vi "纳清蓝绿藻电极校准.vi"() -> ()   [LabVIEW 2016, in "斯坦道多参数.lvlib"]
uses:
  <vilib>/Utility/miscctls.llb/LVPointTypeDef.ctl
  <vilib>/Utility/miscctls.llb/LVPositionTypeDef.ctl
  <vilib>/Analysis/NI_AALBase.lvlib
panel:
  out "第三点信号值":dbl
  out "第二点信号值":dbl
  out "第一点信号值":dbl
  out "报警信息":string
  out "通讯状态":string
  out "第三点校准值":dbl
  out "标液3":sgl
  out "第二点校准值":dbl
  out "第一点校准值":dbl
  in  "校准停止":bool
  in  "校准启动":bool
  in  "校准模式":enum16{"两点校准", "单点校准", "三点校准"}(ring)=enum."单点校准"
  out "最小值":sgl format="%#.2f"
  out "最大值":sgl format="%#.2f"
  out "波形图表":u16(graph) caption="历史曲线"
  out "mean":dbl caption="均值" format="%#.2f"
  out "standard deviation":dbl caption="标准差" format="%#.2f"
  out "变异系数":dbl format="%#.6f"
  out "测量值":sgl format="%#.2f"
  out "提示":string
  out "标液2":sgl
  out "标液1":sgl
  out "原始光强数值":u16 caption="信号值"
  out "温度":dbl format="%#.2f"
  # "藻密度电极设定"
  # "℃"
  # "cells/mL"
  # "请选择校准模式:"
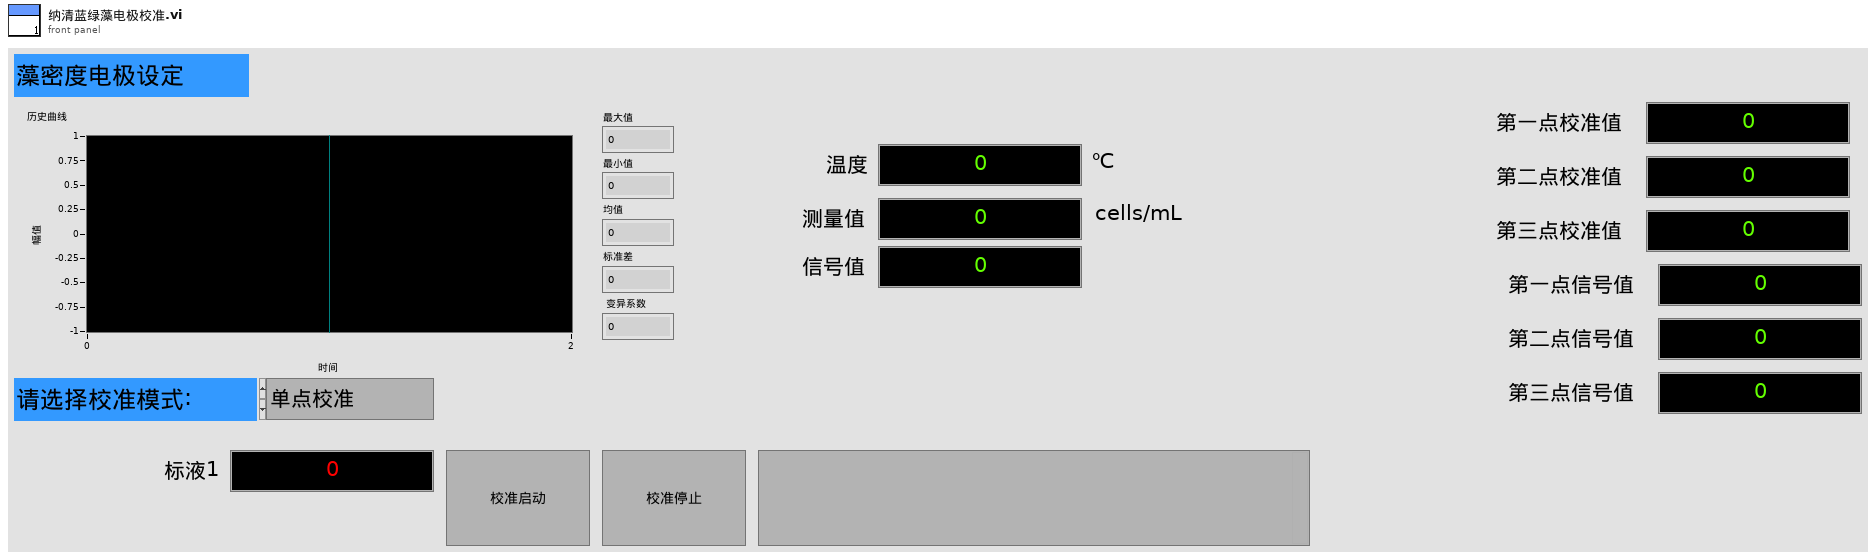
[diagram p1: front panel]
types:
  T1 = typedef "LVPointTypeDef.ctl" = cluster{"Horizontal":i16, "Vertical":i16}
  T2 = cluster{"报警码":u16, "蓝绿藻":sgl, "温度数据":sgl, "原始光强数值":u16, "0X0006_NC":u16, "平均次数":u16, "清扫模式":u16, "清扫次数":u16, "清扫间隔分钟":u16, "0X000B_NC":string, "产品名称":string, "序列号":string, "硬件版本":string, "软件版本":string, "通讯地址":u16, "波特率":u16, "设备类型":u16, "0X0026_NC":string, "0X0030_NC":u16, "第一点原始光强":u16, "第一点校准数据":sgl, "第二点原始光强":u16, "第二点校准数据":sgl, "第三点原始光强":u16, "第三点校准数据":sgl, "探头校准命令":u16, "温度校准参数":sgl, "温度校准命令":u16}
  T3 = typedef "LVPositionTypeDef.ctl" = cluster{"Left":i32, "Top":i32}
  T4 = enum8{"Enabled", "Disabled", "Disabled and Grayed Out"}
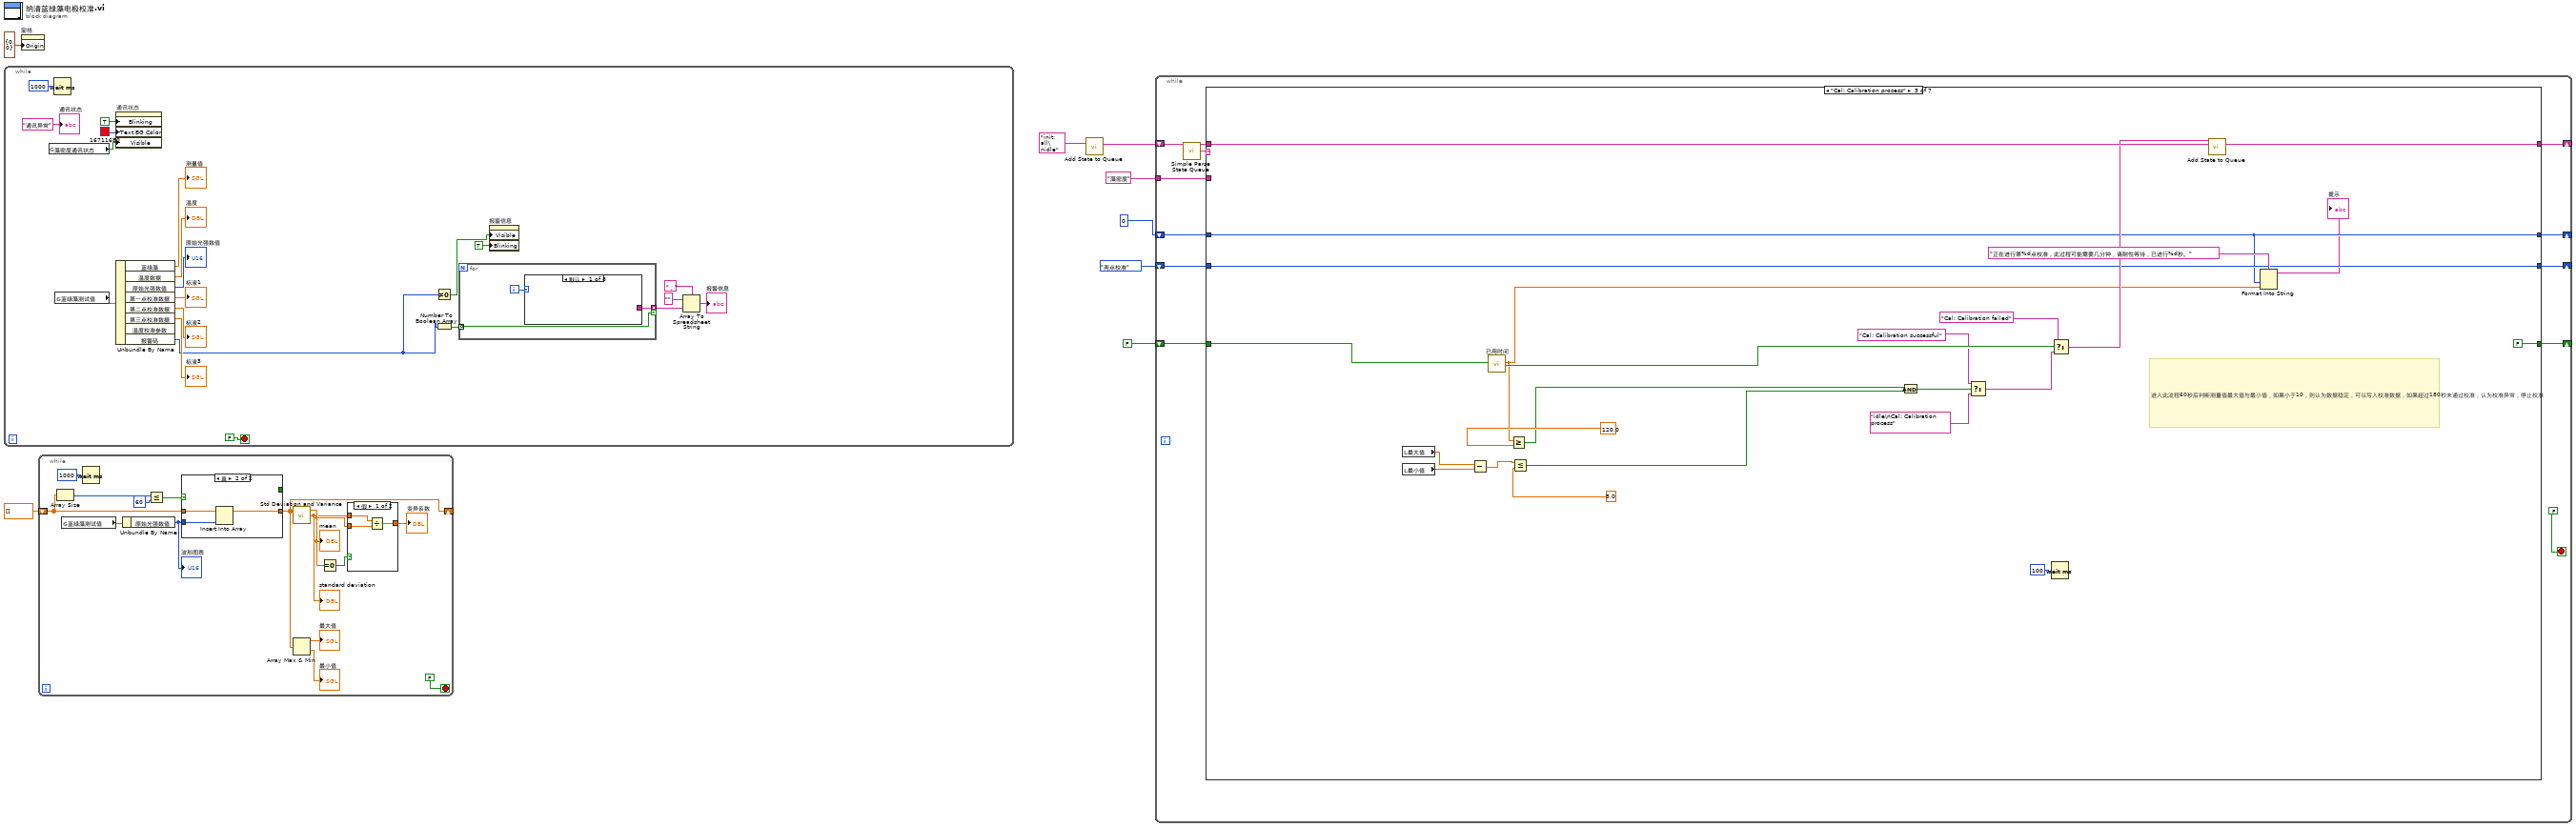
[diagram p0: block diagram]
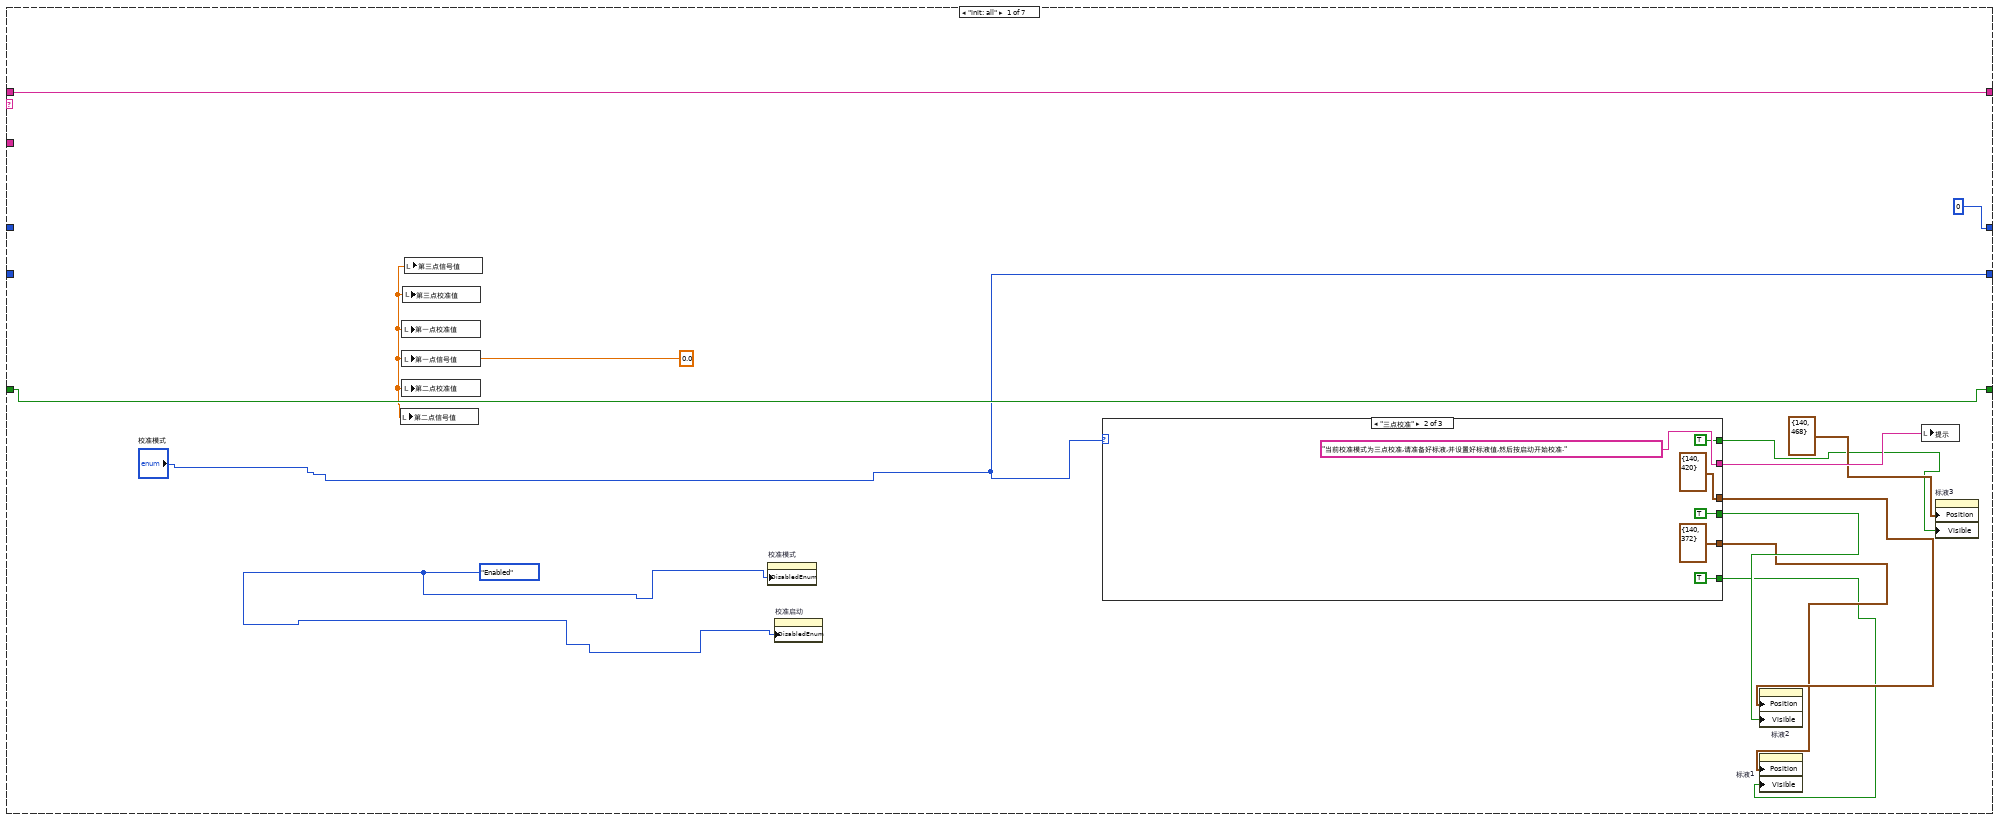
[diagram p2: hidden frame]
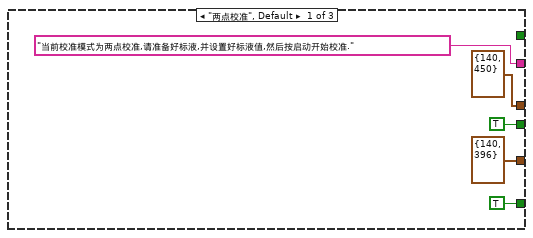
[diagram p3: hidden frame]
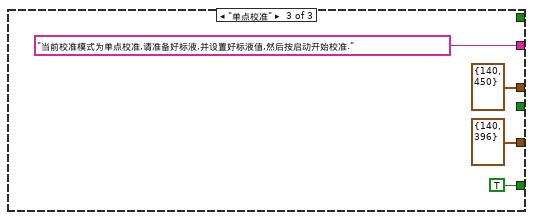
[diagram p4: hidden frame]
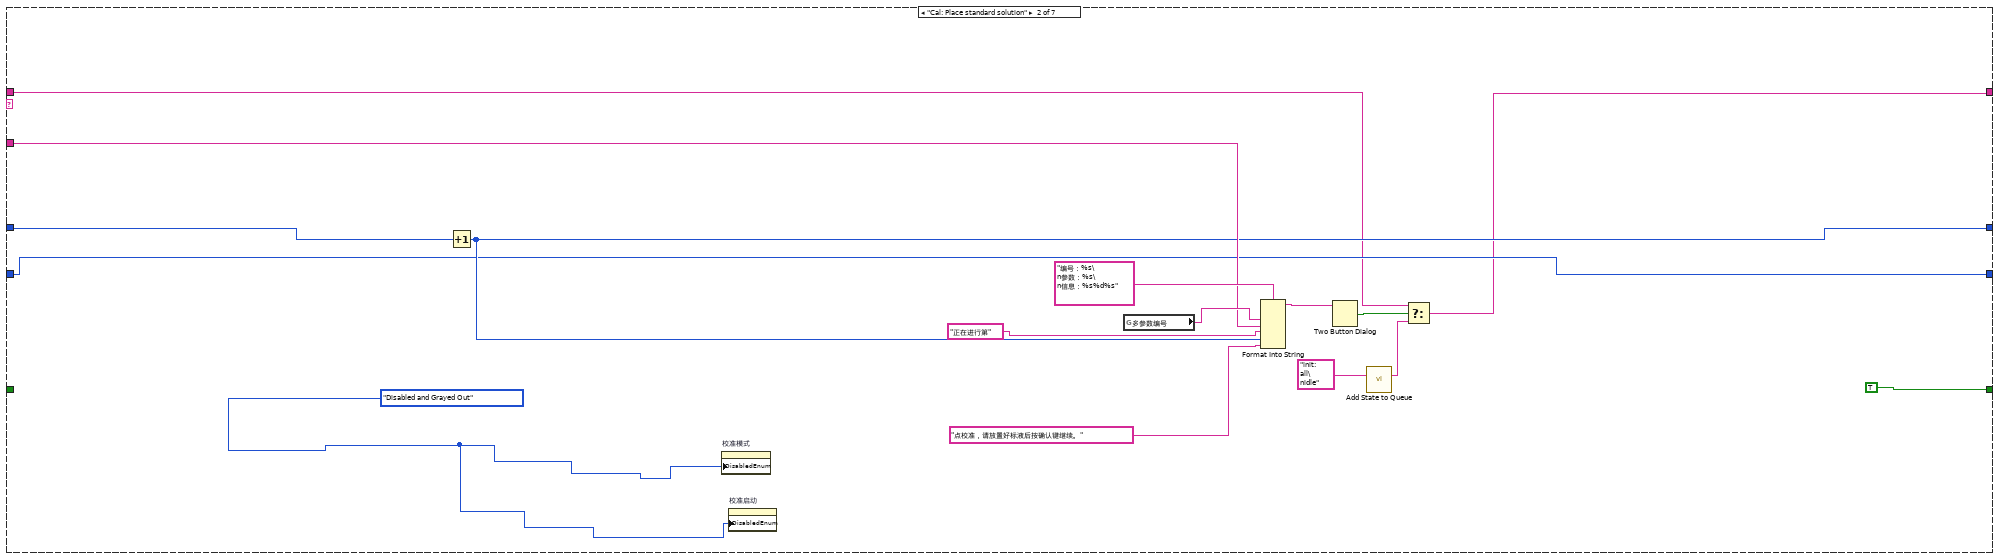
[diagram p5: hidden frame]
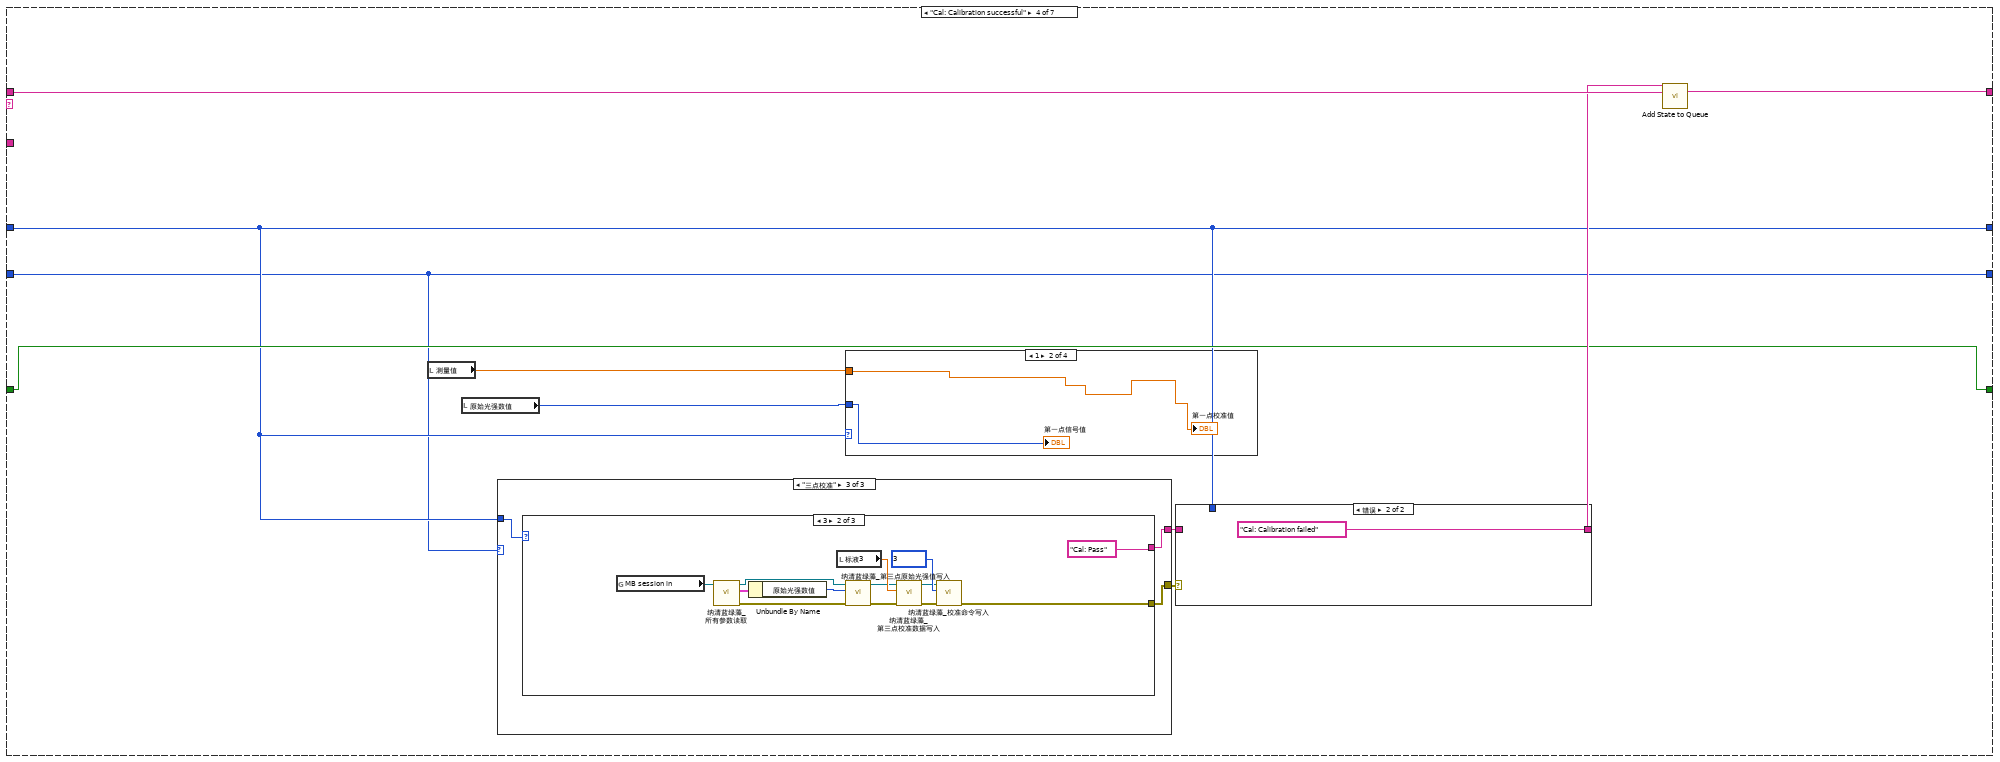
[diagram p6: hidden frame]
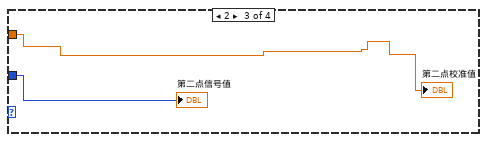
[diagram p8: hidden frame]
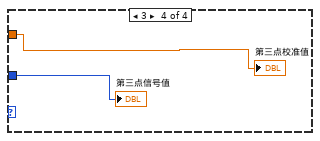
[diagram p9: hidden frame]
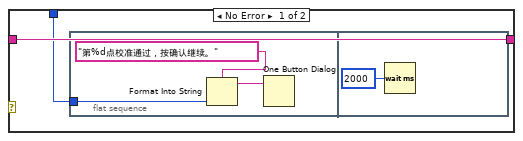
[diagram p10: hidden frame]
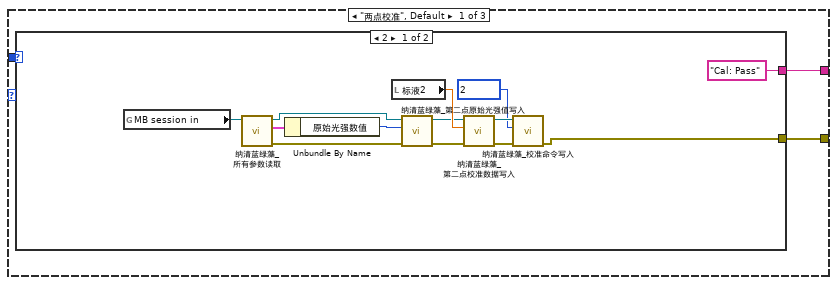
[diagram p11: hidden frame]
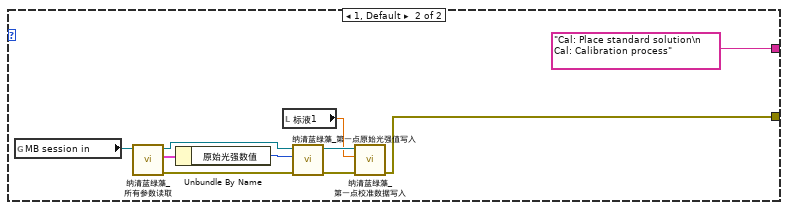
[diagram p12: hidden frame]
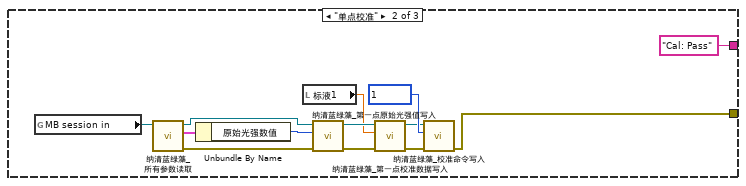
[diagram p13: hidden frame]
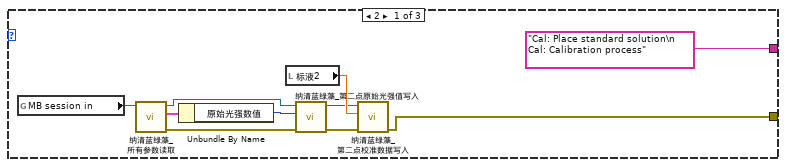
[diagram p14: hidden frame]
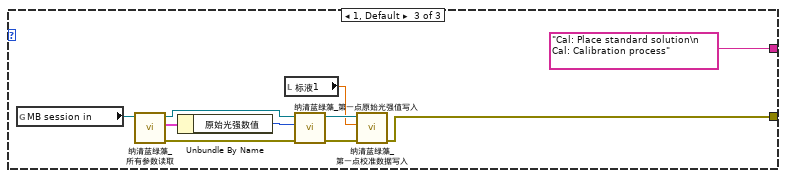
[diagram p15: hidden frame]
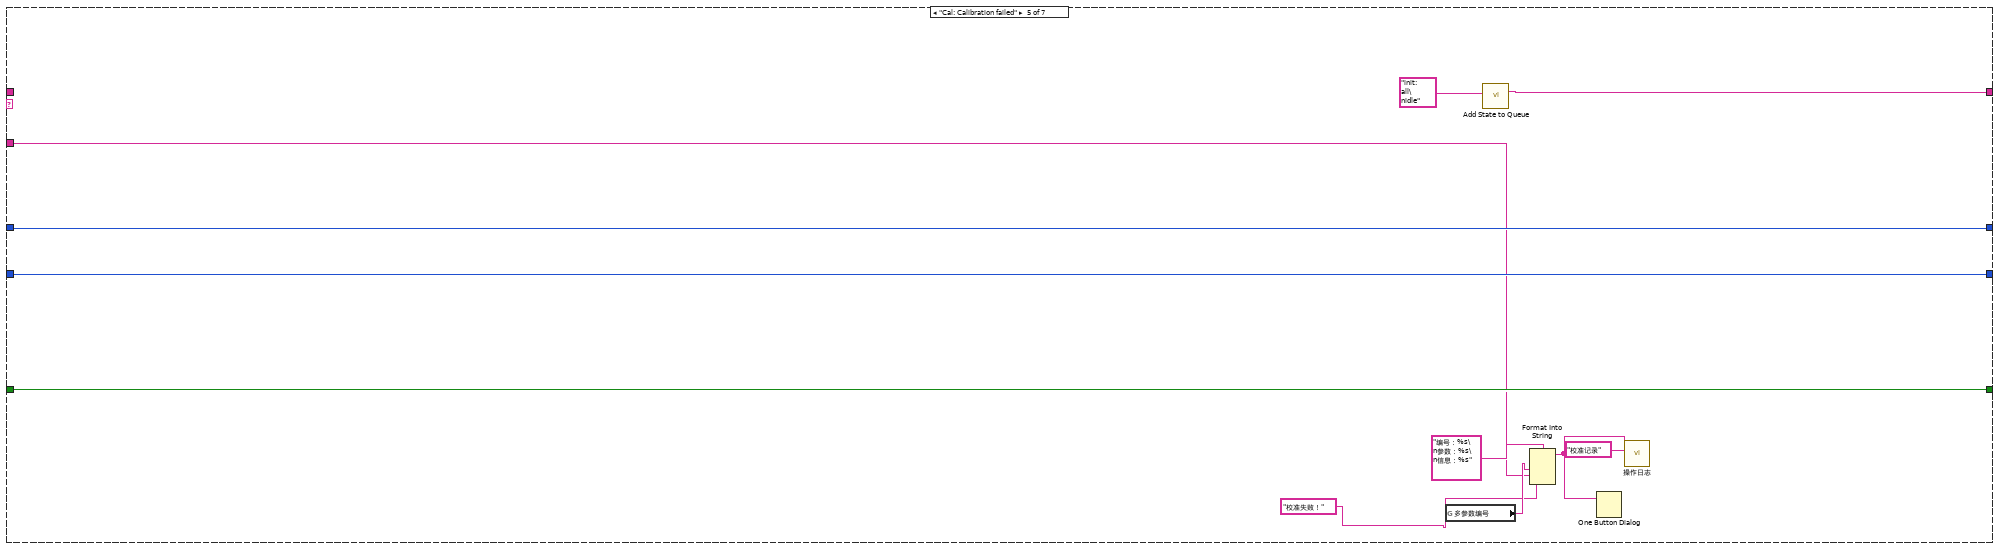
[diagram p16: hidden frame]
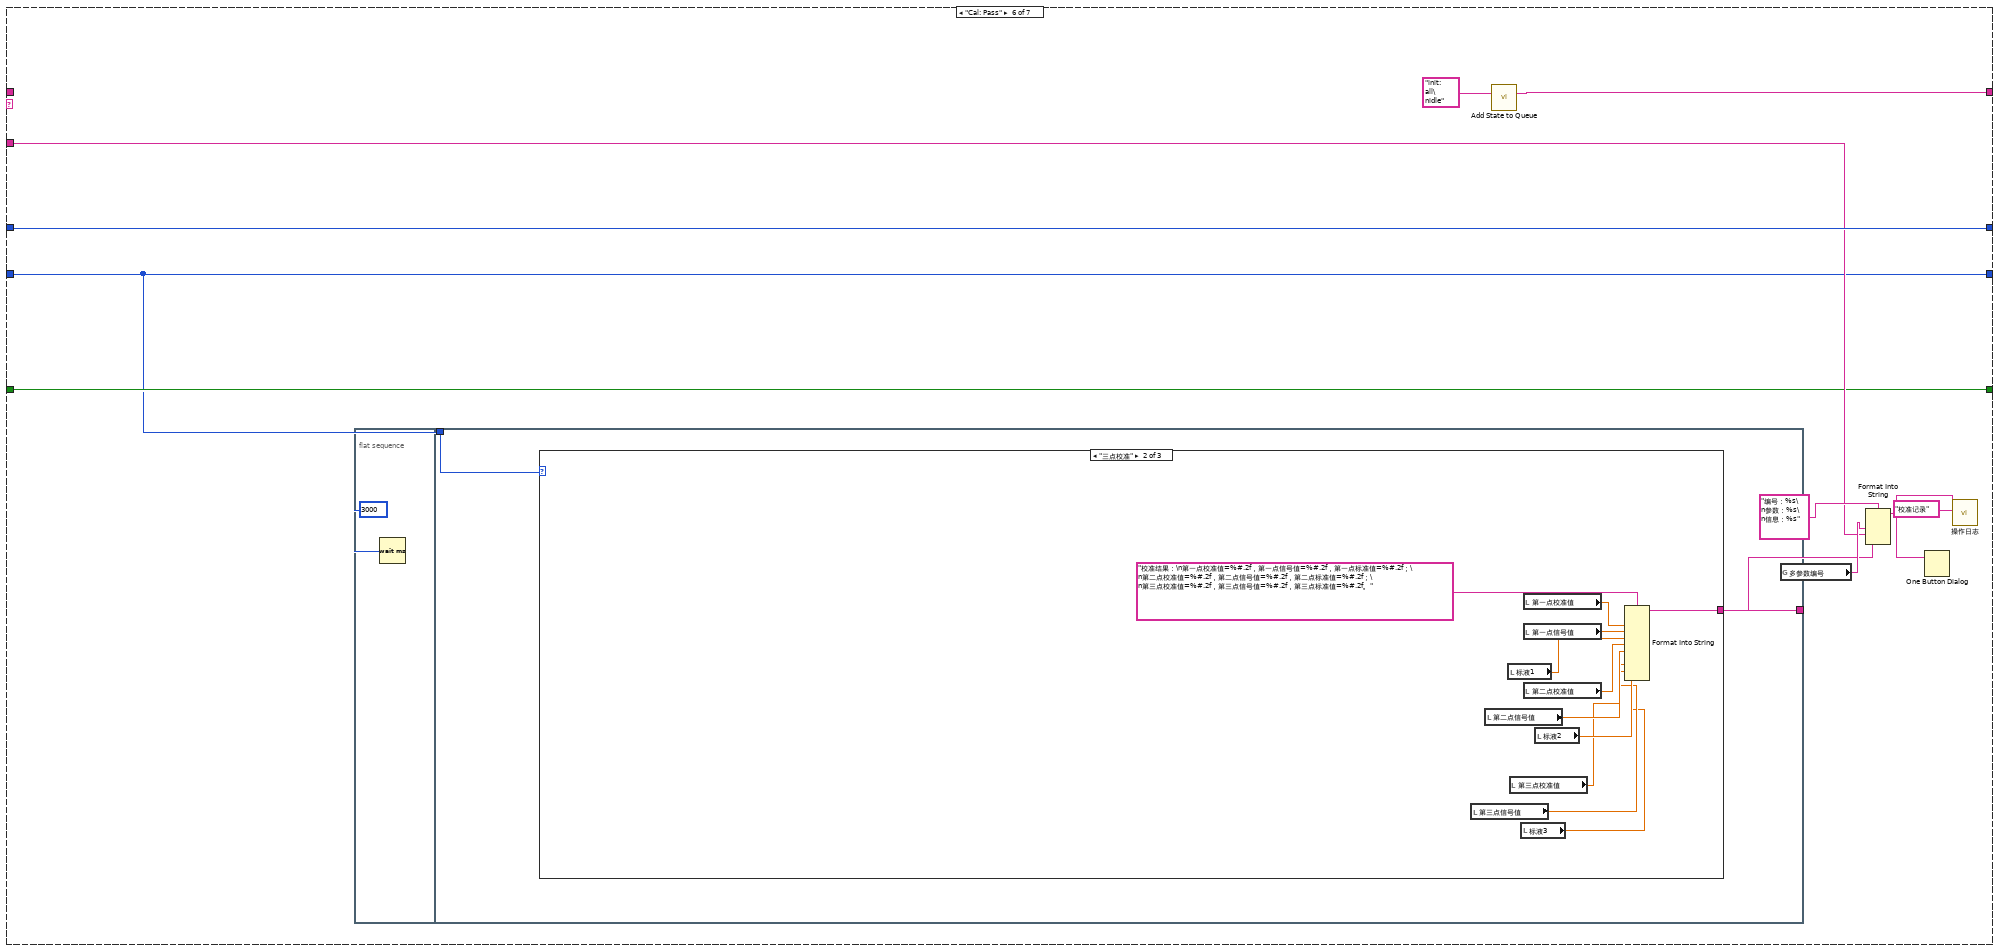
[diagram p17: hidden frame]
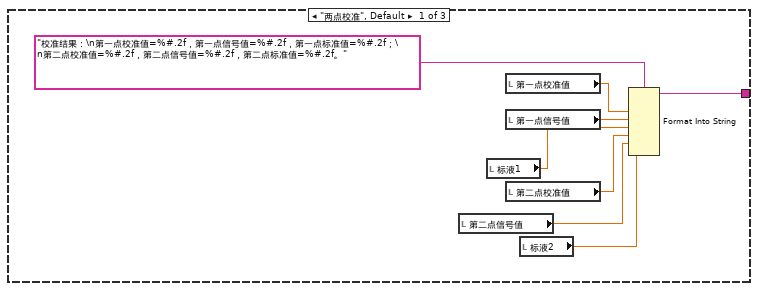
[diagram p18: hidden frame]
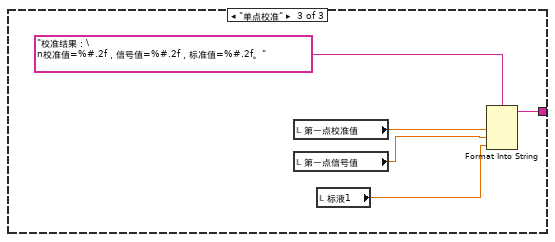
[diagram p19: hidden frame]
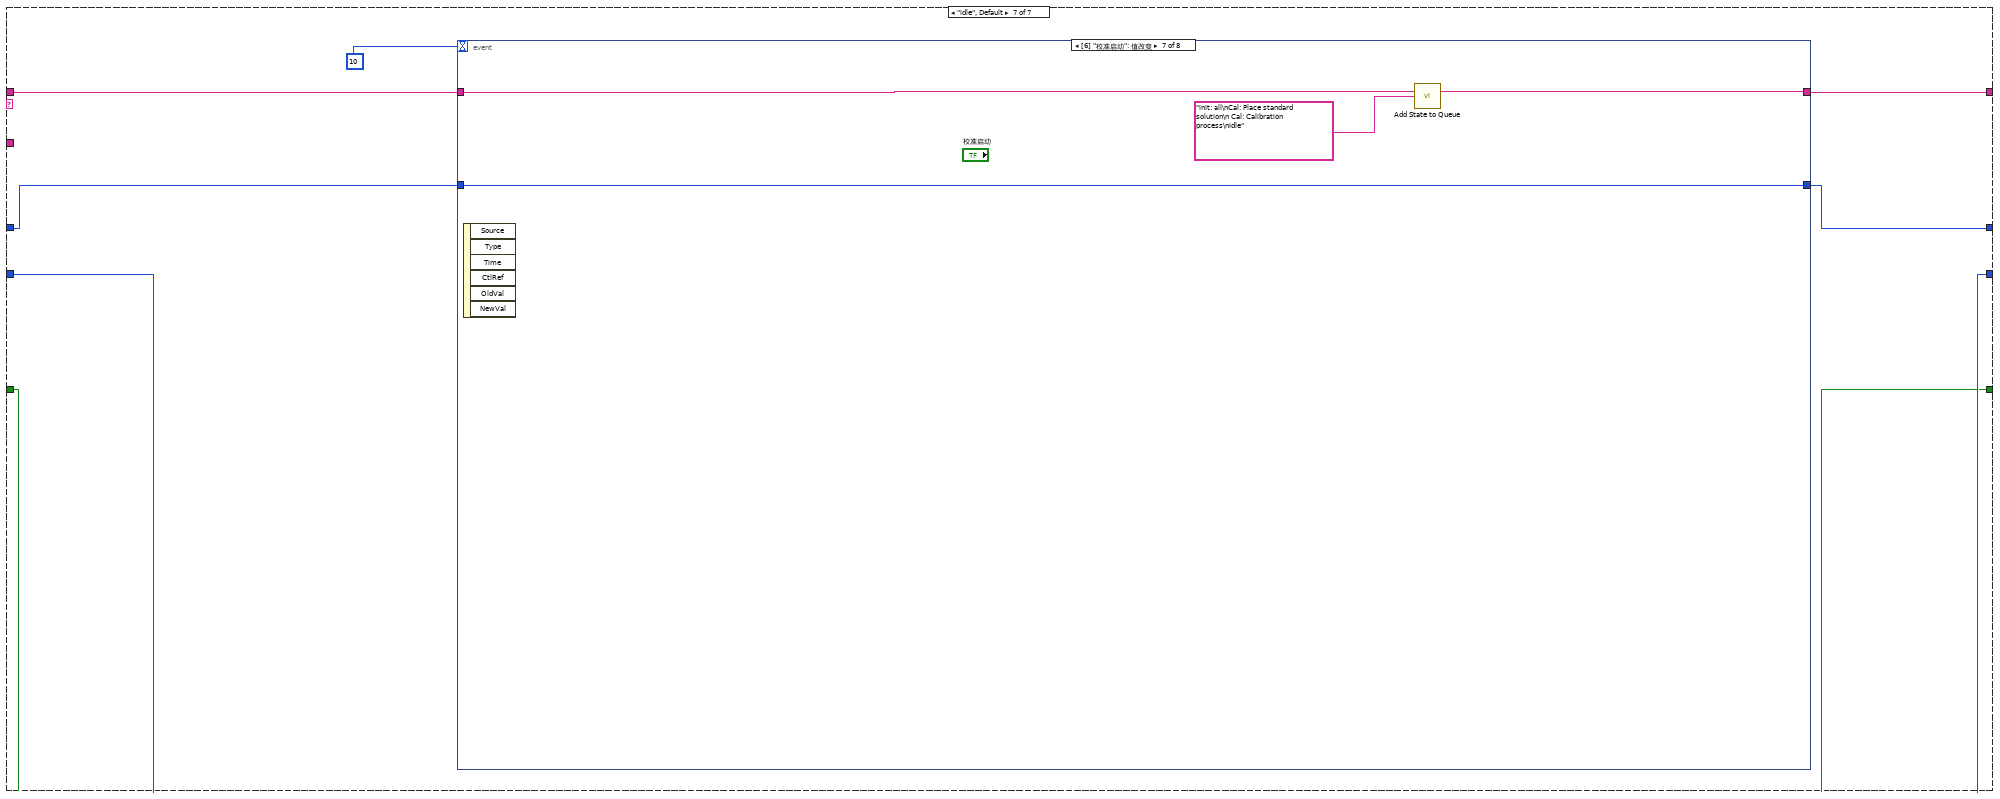
[diagram p20: hidden frame]
diagram:
  n1 = while {
    stop <- FALSE stop-if-true
    n2 = global read "多参数全局变量.vi" "藻密度通讯状态"() -> (w17:bool)
    n3 = Wait (ms)(milliseconds to wait=u32 1000 ("等待时间（毫秒）")) -> ()  [unwired: 1 out]
    n4 = global read "纳清过程全局变量.vi" "蓝绿藻测试值"() -> (w27:T2)
    n5 = property on="通讯状态" class="Str"("Blinking"=TRUE ("闪烁"), "Text.BG Color"=u32 16711680, "Visible"=w17) -> ()  [unwired: 2 in, 2 out]
    n6 = Unbundle By Name(w27) -> ("蓝绿藻"=→"测量值":sgl, "温度数据"=→"温度":sgl, "原始光强数值"=→"原始光强数值":u16, "第一点校准数据"=→"标液1":sgl, "第二点校准数据"=→"标液2":sgl, "第三点校准数据"=→"标液3":sgl, "报警码"=w9:u16)  [unwired: 1 out]
    n7 = Not Equal To 0?(x=w9) -> (x != 0?=w11:bool)
    n8 = Number To Boolean Array(number=w9) -> (Boolean array=w16:bool[])
    n9 = for {
      tunnel: w16 -> [w30] mode=indexing
      tunnel: [w31] -> w15 mode=indexing if=w30
      i -> [w32]
      n10 = case shown="默认" w32 {
        tunnel: [_ "测量值超量程" "温度超量程" "光强信号超范围" "清扫中" "温度传感器故障" "电极故障" "内部电压基准故障"] -> w31
        frame Default {
        }
        frame 0 {
        }
        frame 2 {
        }
        frame 3 {
        }
        frame 4 {
        }
        frame 8 {
        }
        frame 9 {
        }
        frame 10 {
        }
      }
    }
    n11 = property on="报警信息" class="Str"("Visible"=w11, "Blinking"=TRUE ("闪烁")) -> ()  [unwired: 2 in, 2 out]
    n12 = Array To Spreadsheet String(delimiter (Tab)="；" ("分隔符(Tab)"), array=w15, 3:"" ("格式字符串")) -> (spreadsheet string=→"报警信息":string)
    "通讯状态" <- "通讯异常" ("当前串口")
  }
  n13 = property on="窗格" class="Pane"("Origin"=T1 {"Horizontal"=0, "Vertical"=0} ("原点")) -> ()  [unwired: 2 in, 2 out]
  n14 = while {
    shift-right: [w44] -> _
    shift-left: sgl[] [] -> [w50]
    stop <- FALSE stop-if-true
    n15 = Array Size(array=w50) -> (size(s)=w52:i32)
    n16 = global read "纳清过程全局变量.vi" "蓝绿藻测试值"() -> (w40:T2)
    n17 = Wait (ms)(milliseconds to wait=u32 1000 ("等待时间（毫秒）")) -> ()  [unwired: 1 out]
    n18 = Unbundle By Name(w40) -> ("原始光强数值"=w41:u16)
    "波形图表" <- w41
    n19 = Less Or Equal?(x=w52, y=60) -> (x <= y?=w51:bool)
    n20 = case shown="真" w51 {
      tunnel: w50 -> [w63 w66]
      tunnel: w41 -> [w61 w65]
      tunnel: [w59 w64] -> w44
      tunnel: [TRUE _] -> _
      frame False {
        n21 = Replace Array Subset(array=w63, new element=w61) -> (w62:sgl[])  [unwired: 1 in]
        n22 = Rotate 1D Array(1:w62, 2:-1 ("n")) -> (0:w59:sgl[])
      }
      frame True {
        n23 = Insert Into Array(array=w66, new element=w65) -> (w64:sgl[])  [unwired: 1 in]
      }
    }
    n24 = call <vilib>:"Std Deviation and Variance.vi"("X"=w44) -> ("mean"=w48:dbl, "standard deviation"=w47:dbl)  [unwired: 1 in, 1 out]
    "mean" <- w48
    "standard deviation" <- w47
    n25 = Array Max & Min(array=w44) -> (max value=→"最大值":sgl, min value=→"最小值":sgl)  [unwired: 2 out]
    n26 = Equal To 0?(x=w48) -> (x = 0?=w49:bool)
    n27 = case shown="假" w49 {
      tunnel: w47 -> [w57 _]
      tunnel: [w56 _] -> w46
      tunnel: w48 -> [w55 _]
      frame False {
        n28 = Divide(x=w57, y=w55) -> (x/y=w56:dbl)
      }
      frame True {
      }
    }
    "变异系数" <- w46
  }
  n29 = call "Add State to Queue.vi"("State(s) In (\"\")"="init: all\nidle" ("State(s) In (\"\")")) -> ("States Out"=w5:string)  [unwired: 14 in]
  n30 = while {
    shift-right: [w74] -> _
    shift-left: w5 -> [w78]
    shift-right: [w71] -> _
    shift-left: 0 -> [w73]
    tunnel: "藻密度" ("State(s) In (\"\")") -> [w72]
    shift-right: [w69] -> _
    shift-left: enum16{"两点校准", "单点校准", "三点校准"}."两点校准" ("校准模式") -> [w70]
    shift-right: [w67] -> _
    shift-left: FALSE -> [w68]
    stop <- FALSE stop-if-true
    n31 = call "Simple Parse State Queue.vi"("State Queue"=w78) -> ("Remain States"=w75:string, "Next State"=w76:string)  [unwired: 13 in]
    n32 = case shown="\"Cal: Calibration process\"" w76 {
      tunnel: w75 -> [w91 w109 w141 w154 _ _ w300]
      tunnel: [w91 w108 w140 w153 w252 w256 w299] -> w74
      tunnel: w73 -> [_ w118 w125 w148 w255 w266 w297]
      tunnel: w72 -> [_ w119 _ _ w245 w262 _]
      tunnel: [0 w116 w125 w148 w255 w266 w298] -> w71
      tunnel: w70 -> [_ w115 w126 w147 w254 w258 w296]
      tunnel: ["校准模式" w115 w126 w147 w254 w258 w296] -> w69
      tunnel: w68 -> [w89 _ w128 w149 w253 w261 w294]
      tunnel: [w89 TRUE FALSE w149 w253 w261 w294] -> w67
      frame "init: all" {
        w85 = T4."Enabled" ("禁用")
        w88 = 0.0 ("第一点校准值")
        n33 = local write "第二点信号值"(w88) -> ()
        n34 = local write "第一点校准值"(w88) -> ()
        n35 = local write "第一点信号值"(w88) -> ()
        n36 = local write "第二点校准值"(w88) -> ()
        n37 = local write "第三点校准值"(w88) -> ()
        n38 = local write "第三点信号值"(w88) -> ()
        n39 = property on="校准模式" class="Enum (严格)"("DisabledEnum"=w85) -> ()  [unwired: 2 in, 2 out]
        n40 = property on="校准启动" class="Bool"("DisabledEnum"=w85) -> ()  [unwired: 2 in, 2 out]
        n41 = case shown="\"三点校准\"" "校准模式" {
          tunnel: ["当前校准模式为两点校准,请准备好标液,并设置好标液值,然后按启动开始校准." ("提示") "当前校准模式为三点校准,请准备好标液,并设置好标液值,然后按启动开始校准." ("提示") "当前校准模式为单点校准,请准备好标液,并设置好标液值,然后按启动开始校准." ("提示")] -> w87
          tunnel: [TRUE ("可见") TRUE ("可见") _] -> w81
          tunnel: [T3 {"Left"=140, "Top"=396} ("位置") T3 {"Left"=140, "Top"=372} ("位置") T3 {"Left"=140, "Top"=396} ("位置")] -> w80
          tunnel: [T3 {"Left"=140, "Top"=450} ("位置 2") T3 {"Left"=140, "Top"=420} ("位置 2") T3 {"Left"=140, "Top"=450} ("位置 2")] -> w82
          tunnel: [_ TRUE ("可见") _] -> w83
          tunnel: [TRUE ("可见") TRUE ("可见") TRUE ("可见")] -> w79
          frame "两点校准", Default {
          }
          frame "三点校准" {
          }
          frame "单点校准" {
          }
        }
        n42 = property on="标液2" class="DigNum (严格)"("Position"=w82, "Visible"=w81) -> ()  [unwired: 2 in, 2 out]
        n43 = property on="标液1" class="DigNum (严格)"("Position"=w80, "Visible"=w79) -> ()  [unwired: 2 in, 2 out]
        n44 = local write "提示"(w87) -> ()
        n45 = property on="标液3" class="DigNum (严格)"("Position"=T3 {"Left"=140, "Top"=468} ("位置 3"), "Visible"=w83) -> ()  [unwired: 2 in, 2 out]
      }
      frame "Cal: Place standard solution" {
        w107 = T4."Disabled and Grayed Out" ("禁用")
        n46 = Increment(x=w118) -> (x+1=w116:i32)
        n47 = property on="校准模式" class="Enum (严格)"("DisabledEnum"=w107) -> ()  [unwired: 2 in, 2 out]
        n48 = property on="校准启动" class="Bool"("DisabledEnum"=w107) -> ()  [unwired: 2 in, 2 out]
        n49 = global read "多参数全局变量.vi" "多参数编号"() -> (w121:string)
        n50 = Format Into String(format string="编号：%s\n参数：%s\n信息：%s%d%s" ("格式字符串"), w121, w119, "正在进行第" ("消息"), w116, "点校准，请放置好标液后按确认键继续。" ("消息")) -> (resulting string=w113:string)  [unwired: 2 in, 1 out]
        n51 = Two Button Dialog(message=w113) -> (T button?=w112:bool)  [unwired: 2 in]
        n52 = call "Add State to Queue.vi"("State(s) In (\"\")"="init: all\nidle" ("State(s) In (\"\")")) -> ("States Out"=w110:string)  [unwired: 14 in]
        n53 = Select(t=w109, s=w112, f=w110) -> (s? t:f=w108:string)
      }
      frame "Cal: Calibration process" {
        # "进入此流程60秒后判断测量值最大值与最小值，如果小于10，则认为数据稳定，可以写入校准数据，如果超过180秒未通过校准，认为校准异常，停止校准"
        n54 = local read "最大值"() -> (w145:sgl)
        n55 = local read "最小值"() -> (w144:sgl)
        n56 = Subtract(x=w145, y=w144) -> (x-y=w146:sgl)
        n57 = call "已用时间"("Reset"=w128) -> ("Elapsed Time (s)"=w124:dbl, "Time has Elapsed"=w142:bool)  [unwired: 11 in, 6 out]
        n58 = Greater Or Equal?(x=w124, y=120.0) -> (x >= y?=w137:bool)
        n59 = Less Or Equal?(x=w146, y=5.0) -> (x <= y?=w133:bool)
        n60 = And(x=w137, y=w133) -> (x .and. y?=w134:bool)
        n61 = Select(t="Cal: Calibration successful" ("State(s) In (\"\")"), s=w134, f="idle\nCal: Calibration process" ("State(s) In (\"\")")) -> (s? t:f=w132:string)
        n62 = Wait (ms)(milliseconds to wait=u32 100 ("等待时间（毫秒）")) -> ()  [unwired: 1 out]
        n63 = Select(t="Cal: Calibration failed" ("State(s) In (\"\")"), s=w142, f=w132) -> (s? t:f=w131:string)
        n64 = call "Add State to Queue.vi"("State(s) In Front (\"\")"=w131, "State(s) In (\"\")"=w141) -> ("States Out"=w140:string)  [unwired: 13 in]
        n65 = Format Into String(format string="正在进行第%d点校准，此过程可能需要几分钟，请耐性等待，已进行%d秒。" ("格式字符串"), w125, w124) -> (resulting string=→"提示":string)  [unwired: 2 in, 1 out]
      }
      frame "Cal: Calibration successful" {
        n66 = local read "测量值"() -> (w150:sgl)
        n67 = local read "原始光强数值"() -> (w151:u16)
        n68 = case shown="\"三点校准\"" w147 {
          tunnel: [w172 w196 w209] -> w156
          tunnel: [w171 "Cal: Pass" ("State(s) In (\"\")") w210] -> w155
          tunnel: w148 -> [w170 _ w211]
          frame "两点校准", Default {
            n69 = case shown="2" w170 {
              tunnel: [w173 w186] -> w172
              tunnel: ["Cal: Pass" ("State(s) In (\"\")") "Cal: Place standard solution\n Cal: Calibration process" ("State(s) In (\"\")")] -> w171
              frame 2 {
                n70 = global read "多参数全局变量.vi" "MB session in"() -> (w177:refnum<class "MB_Master.lvclass">)
                n71 = call "纳清蓝绿藻_所有参数读取.vi"("MB session in"=w177) -> ("error out"=w175:errorcluster, "输出值"=w178:T2, "MB session out"=w176:refnum<class "MB_Master.lvclass">)  [unwired: 8 in]
                n72 = Unbundle By Name(w178) -> ("原始光强数值"=w179:u16)
                n73 = local read "标液2"() -> (w184:sgl)
                n74 = call "纳清蓝绿藻_第二点原始光强值写入.vi"("error in (no error)"=w175, "数值"=w179, "MB session in"=w176) -> ("error out"=w180:errorcluster, "MB session out"=w181:refnum<class "MB_Master.lvclass">)  [unwired: 7 in]
                n75 = call "纳清蓝绿藻_第二点校准数据写入.vi"("error in (no error)"=w180, "数值"=w184, "MB session in"=w181) -> ("error out"=w182:errorcluster, "MB session out"=w183:refnum<class "MB_Master.lvclass">)  [unwired: 7 in]
                n76 = call "纳清蓝绿藻_校准命令写入.vi"("error in (no error)"=w182, "数值"=u16 2 ("starting address"), "MB session in"=w183) -> ("error out"=w173:errorcluster)  [unwired: 7 in, 1 out]
              }
              frame 1, Default {
                n77 = global read "多参数全局变量.vi" "MB session in"() -> (w192:refnum<class "MB_Master.lvclass">)
                n78 = call "纳清蓝绿藻_所有参数读取.vi"("MB session in"=w192) -> ("error out"=w194:errorcluster, "输出值"=w191:T2, "MB session out"=w193:refnum<class "MB_Master.lvclass">)  [unwired: 8 in]
                n79 = Unbundle By Name(w191) -> ("原始光强数值"=w190:u16)
                n80 = local read "标液1"() -> (w187:sgl)
                n81 = call "纳清蓝绿藻_第一点原始光强值写入.vi"("error in (no error)"=w194, "数值"=w190, "MB session in"=w193) -> ("error out"=w189:errorcluster, "MB session out"=w188:refnum<class "MB_Master.lvclass">)  [unwired: 7 in]
                n82 = call "纳清蓝绿藻_第一点校准数据写入.vi"("error in (no error)"=w189, "数值"=w187, "MB session in"=w188) -> ("error out"=w186:errorcluster)  [unwired: 7 in, 1 out]
              }
            }
          }
          frame "单点校准" {
            n83 = global read "多参数全局变量.vi" "MB session in"() -> (w204:refnum<class "MB_Master.lvclass">)
            n84 = call "纳清蓝绿藻_所有参数读取.vi"("MB session in"=w204) -> ("error out"=w206:errorcluster, "输出值"=w203:T2, "MB session out"=w205:refnum<class "MB_Master.lvclass">)  [unwired: 8 in]
            n85 = Unbundle By Name(w203) -> ("原始光强数值"=w202:u16)
            n86 = local read "标液1"() -> (w197:sgl)
            n87 = call "纳清蓝绿藻_第一点原始光强值写入.vi"("error in (no error)"=w206, "数值"=w202, "MB session in"=w205) -> ("error out"=w201:errorcluster, "MB session out"=w200:refnum<class "MB_Master.lvclass">)  [unwired: 7 in]
            n88 = call "纳清蓝绿藻_第一点校准数据写入.vi"("error in (no error)"=w201, "数值"=w197, "MB session in"=w200) -> ("error out"=w199:errorcluster, "MB session out"=w198:refnum<class "MB_Master.lvclass">)  [unwired: 7 in]
            n89 = call "纳清蓝绿藻_校准命令写入.vi"("error in (no error)"=w199, "数值"=u16 1 ("starting address"), "MB session in"=w198) -> ("error out"=w196:errorcluster)  [unwired: 7 in, 1 out]
          }
          frame "三点校准" {
            n90 = case shown="3" w211 {
              tunnel: [w212 w222 w235] -> w209
              tunnel: ["Cal: Place standard solution\n Cal: Calibration process" ("State(s) In (\"\")") "Cal: Pass" ("State(s) In (\"\")") "Cal: Place standard solution\n Cal: Calibration process" ("State(s) In (\"\")")] -> w210
              frame 2 {
                n91 = global read "多参数全局变量.vi" "MB session in"() -> (w215:refnum<class "MB_Master.lvclass">)
                n92 = call "纳清蓝绿藻_所有参数读取.vi"("MB session in"=w215) -> ("error out"=w213:errorcluster, "输出值"=w216:T2, "MB session out"=w214:refnum<class "MB_Master.lvclass">)  [unwired: 8 in]
                n93 = Unbundle By Name(w216) -> ("原始光强数值"=w217:u16)
                n94 = local read "标液2"() -> (w220:sgl)
                n95 = call "纳清蓝绿藻_第二点原始光强值写入.vi"("error in (no error)"=w213, "数值"=w217, "MB session in"=w214) -> ("error out"=w218:errorcluster, "MB session out"=w219:refnum<class "MB_Master.lvclass">)  [unwired: 7 in]
                n96 = call "纳清蓝绿藻_第二点校准数据写入.vi"("error in (no error)"=w218, "数值"=w220, "MB session in"=w219) -> ("error out"=w212:errorcluster)  [unwired: 7 in, 1 out]
              }
              frame 3 {
                n97 = global read "多参数全局变量.vi" "MB session in"() -> (w225:refnum<class "MB_Master.lvclass">)
                n98 = call "纳清蓝绿藻_所有参数读取.vi"("MB session in"=w225) -> ("error out"=w223:errorcluster, "输出值"=w226:T2, "MB session out"=w224:refnum<class "MB_Master.lvclass">)  [unwired: 8 in]
                n99 = Unbundle By Name(w226) -> ("原始光强数值"=w227:u16)
                n100 = local read "标液3"() -> (w233:sgl)
                n101 = call "纳清蓝绿藻_第三点原始光强值写入.vi"("error in (no error)"=w223, "数值"=w227, "MB session in"=w224) -> ("error out"=w228:errorcluster, "MB session out"=w229:refnum<class "MB_Master.lvclass">)  [unwired: 7 in]
                n102 = call "纳清蓝绿藻_第三点校准数据写入.vi"("error in (no error)"=w228, "数值"=w233, "MB session in"=w229) -> ("error out"=w230:errorcluster, "MB session out"=w231:refnum<class "MB_Master.lvclass">)  [unwired: 7 in]
                n103 = call "纳清蓝绿藻_校准命令写入.vi"("error in (no error)"=w230, "数值"=u16 3 ("starting address"), "MB session in"=w231) -> ("error out"=w222:errorcluster)  [unwired: 7 in, 1 out]
              }
              frame 1, Default {
                n104 = global read "多参数全局变量.vi" "MB session in"() -> (w241:refnum<class "MB_Master.lvclass">)
                n105 = call "纳清蓝绿藻_所有参数读取.vi"("MB session in"=w241) -> ("error out"=w243:errorcluster, "输出值"=w240:T2, "MB session out"=w242:refnum<class "MB_Master.lvclass">)  [unwired: 8 in]
                n106 = Unbundle By Name(w240) -> ("原始光强数值"=w239:u16)
                n107 = local read "标液1"() -> (w236:sgl)
                n108 = call "纳清蓝绿藻_第一点原始光强值写入.vi"("error in (no error)"=w243, "数值"=w239, "MB session in"=w242) -> ("error out"=w238:errorcluster, "MB session out"=w237:refnum<class "MB_Master.lvclass">)  [unwired: 7 in]
                n109 = call "纳清蓝绿藻_第一点校准数据写入.vi"("error in (no error)"=w238, "数值"=w236, "MB session in"=w237) -> ("error out"=w235:errorcluster)  [unwired: 7 in, 1 out]
              }
            }
          }
        }
        n110 = case shown="1" w148 {
          tunnel: w151 -> [_ w158 w160 w162]
          tunnel: w150 -> [_ w157 w159 w161]
          frame 0, Default {
          }
          frame 1 {
            "第一点信号值" <- w158
            "第一点校准值" <- w157
          }
          frame 2 {
            "第二点信号值" <- w160
            "第二点校准值" <- w159
          }
          frame 3 {
            "第三点信号值" <- w162
            "第三点校准值" <- w161
          }
        }
        n111 = case shown="错误" w156 {
          tunnel: w155 -> [w164 _]
          tunnel: [w164 "Cal: Calibration failed" ("State(s) In (\"\")")] -> w152
          tunnel: w148 -> [w163 _]
          frame No Error {
            n112 = flat-sequence {
              tunnel: w163 -> [w165]
              frame #0 {
                n113 = Format Into String(format string="第%d点校准通过，按确认继续。" ("格式字符串"), w165) -> (resulting string=w167:string)  [unwired: 2 in, 1 out]
                n114 = One Button Dialog(message=w167) -> ()  [unwired: 1 in, 1 out]
              }
              frame #1 {
                n115 = Wait (ms)(milliseconds to wait=u32 2000 ("等待时间（毫秒）")) -> ()  [unwired: 1 out]
              }
            }
          }
          frame Error {
          }
        }
        n116 = call "Add State to Queue.vi"("State(s) In Front (\"\")"=w152, "State(s) In (\"\")"=w154) -> ("States Out"=w153:string)  [unwired: 13 in]
      }
      frame "Cal: Calibration failed" {
        n117 = global read "多参数全局变量.vi" "多参数编号"() -> (w248:string)
        n118 = call "Add State to Queue.vi"("State(s) In (\"\")"="init: all\nidle" ("State(s) In (\"\")")) -> ("States Out"=w252:string)  [unwired: 14 in]
        n119 = Format Into String(format string="编号：%s\n参数：%s\n信息：%s" ("格式字符串"), w248, w245, "校准失败！" ("消息")) -> (resulting string=w247:string)  [unwired: 2 in, 1 out]
        n120 = One Button Dialog(message=w247) -> ()  [unwired: 1 in, 1 out]
        n121 = call "操作日志.vi"("table"="校准记录", "日志信息"=w247) -> ()  [unwired: 9 in, 1 out]
      }
      frame "Cal: Pass" {
        n122 = flat-sequence {
          tunnel: [w269] -> w259
          tunnel: w258 -> [w268]
          frame #0 {
            n123 = Wait (ms)(milliseconds to wait=u32 3000 ("等待时间（毫秒）")) -> ()  [unwired: 1 out]
          }
          frame #1 {
            n124 = case shown="\"三点校准\"" w268 {
              tunnel: [w277 w288 w293] -> w269
              frame "两点校准", Default {
                n125 = local read "第二点信号值"() -> (w271:dbl)
                n126 = local read "标液1"() -> (w273:sgl)
                n127 = local read "第一点校准值"() -> (w275:dbl)
                n128 = local read "第一点信号值"() -> (w276:dbl)
                n129 = local read "第二点校准值"() -> (w272:dbl)
                n130 = local read "标液2"() -> (w270:sgl)
                n131 = Format Into String(format string="校准结果：\n第一点校准值=%#.2f，第一点信号值=%#.2f，第一点标准值=%#.2f；\n第二点校准值=%#.2f，第二点信号值=%#.2f，第二点标准值=%#.2f。" ("提示"), w275, w276, w273, w272, w271, w270) -> (resulting string=w277:string)  [unwired: 2 in, 1 out]
              }
              frame "三点校准" {
                n132 = local read "第三点信号值"() -> (w279:dbl)
                n133 = local read "第二点信号值"() -> (w282:dbl)
                n134 = local read "标液1"() -> (w284:sgl)
                n135 = local read "第三点校准值"() -> (w280:dbl)
                n136 = local read "标液3"() -> (w278:sgl)
                n137 = local read "第一点校准值"() -> (w286:dbl)
                n138 = local read "第一点信号值"() -> (w287:dbl)
                n139 = local read "第二点校准值"() -> (w283:dbl)
                n140 = local read "标液2"() -> (w281:sgl)
                n141 = Format Into String(format string="校准结果：\n第一点校准值=%#.2f，第一点信号值=%#.2f，第一点标准值=%#.2f；\n第二点校准值=%#.2f，第二点信号值=%#.2f，第二点标准值=%#.2f；\n第三点校准值=%#.2f，第三点信号值=%#.2f，第三点标准值=%#.2f。" ("提示"), w286, w287, w284, w283, w282, w281, w280, w279, w278) -> (resulting string=w288:string)  [unwired: 2 in, 1 out]
              }
              frame "单点校准" {
                n142 = local read "第一点校准值"() -> (w292:dbl)
                n143 = local read "第一点信号值"() -> (w290:dbl)
                n144 = local read "标液1"() -> (w289:sgl)
                n145 = Format Into String(format string="校准结果：\n校准值=%#.2f，信号值=%#.2f，标准值=%#.2f。" ("提示"), w292, w290, w289) -> (resulting string=w293:string)  [unwired: 2 in, 1 out]
              }
            }
          }
        }
        n146 = call "Add State to Queue.vi"("State(s) In (\"\")"="init: all\nidle" ("State(s) In (\"\")")) -> ("States Out"=w256:string)  [unwired: 14 in]
        n147 = global read "多参数全局变量.vi" "多参数编号"() -> (w263:string)
        n148 = Format Into String(format string="编号：%s\n参数：%s\n信息：%s" ("格式字符串"), w263, w262, w259) -> (resulting string=w260:string)  [unwired: 2 in, 1 out]
        n149 = One Button Dialog(message=w260) -> ()  [unwired: 1 in, 1 out]
        n150 = call "操作日志.vi"("table"="校准记录", "日志信息"=w260) -> ()  [unwired: 9 in, 1 out]
      }
      frame "idle", Default {
        n151 = event shown="[6] \"校准启动\": 值改变" {
          selector: _ -> [_ _ _ _ _ _ _ _]
          dyn-events: _ -> [_ _ _ _ _ _ _ _]
          timeout: 10 -> [_ _ _ _ _ _ _ _]
          tunnel: w300 -> [w303 w307 w310 w317 w322 w327 w335 _]
          tunnel: [w302 w306 w311 w321 w326 w331 w334 w337] -> w299
          tunnel: [w301 w304 w312 w320 w325 w330 w332 w338] -> w298
          tunnel: w297 -> [w301 w304 w312 w320 w325 w330 w332 w338]
          event Timeout {
            n152 = event-data() -> ()  [unwired: 1 in, 3 out]
            n153 = call "Add State to Queue.vi"("State(s) In (\"\")"=w303) -> ("States Out"=w302:string)  [unwired: 14 in]
          }
          event "校准模式": Value Change {
            n154 = event-data() -> ()  [unwired: 1 in, 6 out]
            n155 = call "Add State to Queue.vi"("State(s) In (\"\")"=w307, "State(s) At Back (\"\")"="init: all\nidle" ("State(s) In (\"\")")) -> ("States Out"=w306:string)  [unwired: 13 in]
          }
          event "标液1", "标液2", "标液3": Mouse Down {
            n156 = event-data() -> ("CtlRef"=w309:refnum<vi>)  [unwired: 1 in, 7 out]
            n157 = property class="DigNum (严格)"(reference=w309) -> ("DisabledEnum"=w308:T4)  [unwired: 1 in, 2 out]
            n158 = case shown="\"Enabled\"" w308 {
              tunnel: w309 -> [w316 _]
              frame "Enabled" {
                n159 = property class="DigNum (严格)"(reference=w316) -> (reference out=w313:refnum<vi>, "Value"=w314:sgl)  [unwired: 1 in, 1 out]
                n160 = call "数字键盘.vi"("OldNumber"=w314) -> ("NewNumber"=w315:dbl)  [unwired: 1 in]
                n161 = property class="DigNum (严格)"(reference=w313, "Val(Sgnl)"=w315) -> ()  [unwired: 1 in, 2 out]
              }
              frame "Disabled", Default {
              }
            }
            n162 = call "Add State to Queue.vi"("State(s) In (\"\")"=w310) -> ("States Out"=w311:string)  [unwired: 14 in]
          }
          event "标液1": Value Change {
            n163 = event-data() -> ("NewVal"=w318:sgl)  [unwired: 1 in, 5 out]
            n164 = global read "多参数全局变量.vi" "MB session in"() -> (w319:refnum<class "MB_Master.lvclass">)
            n165 = call "纳清蓝绿藻_第一点校准数据写入.vi"("数值"=w318, "MB session in"=w319) -> ()  [unwired: 8 in, 2 out]
            n166 = call "Add State to Queue.vi"("State(s) In (\"\")"=w317) -> ("States Out"=w321:string)  [unwired: 14 in]
          }
          event "标液2": Value Change {
            n167 = event-data() -> ("NewVal"=w323:sgl)  [unwired: 1 in, 5 out]
            n168 = global read "多参数全局变量.vi" "MB session in"() -> (w324:refnum<class "MB_Master.lvclass">)
            n169 = call "纳清蓝绿藻_第二点校准数据写入.vi"("数值"=w323, "MB session in"=w324) -> ()  [unwired: 8 in, 2 out]
            n170 = call "Add State to Queue.vi"("State(s) In (\"\")"=w322) -> ("States Out"=w326:string)  [unwired: 14 in]
          }
          event "标液3": Value Change {
            n171 = event-data() -> ("NewVal"=w328:sgl)  [unwired: 1 in, 5 out]
            n172 = global read "多参数全局变量.vi" "MB session in"() -> (w329:refnum<class "MB_Master.lvclass">)
            n173 = call "纳清蓝绿藻_第三点校准数据写入.vi"("数值"=w328, "MB session in"=w329) -> ()  [unwired: 8 in, 2 out]
            n174 = call "Add State to Queue.vi"("State(s) In (\"\")"=w327) -> ("States Out"=w331:string)  [unwired: 14 in]
          }
          event "校准启动": Value Change {
            n175 = event-data() -> ()  [unwired: 1 in, 6 out]
            n176 = call "Add State to Queue.vi"("State(s) In (\"\")"=w335, "State(s) At Back (\"\")"="init: all\nCal: Place standard solution\n Cal: Calibration process\nidle" ("State(s) In (\"\")")) -> ("States Out"=w334:string)  [unwired: 13 in]
          }
          event "校准停止": Value Change {
            n177 = event-data() -> ()  [unwired: 1 in, 6 out]
            n178 = call "Add State to Queue.vi"("State(s) In (\"\")"="init: all\nidle" ("State(s) In (\"\")")) -> ("States Out"=w337:string)  [unwired: 14 in]
          }
        }
      }
    }
  }
